vi "Create Execution Unit.vi"(8 "error in":errorcluster, 10 "Item Ref":T2=18446744073709551615 format="%.0x", 11 "Execution Unit Factory Implementation in":refnum<class "Execution Unit Factory.lvclass">) -> (0 "error out":errorcluster, 1 "Asynchronous Execution Units":cluster{"Grouped Execution Units":T1[]}[](array[cluster]) {"Grouped Execution Units"."ReadWrite Channels" format="%.0x"; "Grouped Execution Units"."Outgoing Channels" format="%.0x"; "Grouped Execution Units"."Incoming Channels" format="%.0x"}, 2 "Inline Execution Units":T1[](array[typedef]) {"ReadWrite Channels" format="%.0x"; "Outgoing Channels" format="%.0x"; "Incoming Channels" format="%.0x"}, 3 "Execution Unit Factory Implementation out":refnum<class "Execution Unit Factory.lvclass">)   [LabVIEW 2020, in "Ballard ARINC 429 Engine.lvlib" / "Implementation.lvlib" / "Execution Unit Factory.lvclass"]
uses:
  Execution Unit Factory.lvclass
  <vilib>/NI VeriStand/Custom Device API/Custom Device Item Ref.ctl
  Interfaces/Controls/Execution Unit Information.ctl
  Interfaces/Execution Unit/Execution Unit.lvclass
  Rx Execution Unit/Rx Execution Unit.lvclass
  C:/git/ni/niveristand-ballard-arinc429-custom-device/Source/Custom Device Support/Engine/Interfaces/Execution Unit/Execution Unit.lvclass
  Tx Acyclic Labels Execution Unit/Tx Acyclic Labels Execution Unit.lvclass
  Tx Scheduled Labels Execution Unit/Tx Scheduled Labels Execution Unit.lvclass
  <vilib>/NI VeriStand/Custom Device API/Custom Device API.lvlib
  Interfaces/Interfaces.lvlib
  System Explorer/Implementation/Implementation.lvlib
  Scripting/Ballard/Ballard ARINC 429 Scripting.lvlib
  Custom Device/Custom Device.lvlib
  C:/git/ni/niveristand-ballard-arinc429-custom-device/Source/Custom Device Support/Engine/Implementation/Execution Unit/Execution Unit.lvclass
  C:/git/ni/niveristand-ballard-arinc429-custom-device/Source/Custom Device Support/Engine/Implementation/Rx Execution Unit/Rx Execution Unit.lvclass
  C:/git/ni/niveristand-ballard-arinc429-custom-device/Source/Custom Device Support/Engine/Implementation/Tx Acyclic Labels Execution Unit/Tx Acyclic Labels Execution Unit.lvclass
  C:/git/ni/niveristand-ballard-arinc429-custom-device/Source/Custom Device Support/Engine/Implementation/Tx Scheduled Labels Execution Unit/Tx Scheduled Labels Execution Unit.lvclass
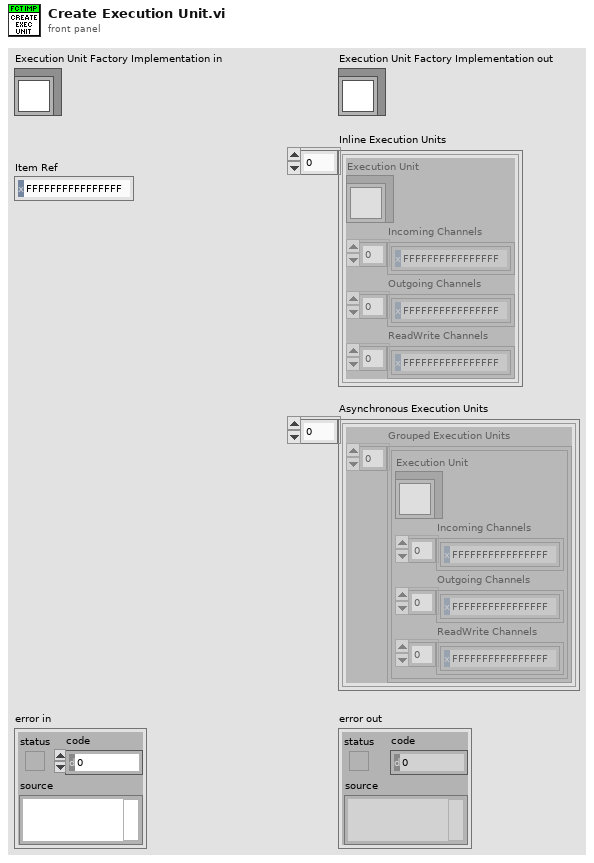
[diagram p1: front panel]
types:
  T1 = typedef "Ballard ARINC 429 Engine.lvlib/Interfaces.lvlib/Execution Unit Information.ctl" = cluster{"Execution Unit":refnum<class "Execution Unit.lvclass">, "Incoming Channels":T2[], "Outgoing Channels":T2[], "ReadWrite Channels":T2[]}
  T2 = typedef "Custom Device API.lvlib/Custom Device Item Ref.ctl" = u64
  T3 = typedef "RT Hardware Channel Settings.ctl" = cluster{"channel #":u16, "channel handle":u64, "labels settings for RT":T4[]}
  T4 = typedef "RT Label Settings.ctl" = cluster{"Name":string, "xmlName":string, "label":T5, "transfer period":u32, "SDI_Enabled":bool, "SDI":u8, "parameter driver data":T6, "transfer type":T9, "has timestamp?":bool, "Label Disable/Trigger Channel Reference":T2, "Message Handle":u64, "Initialized?":bool, "Word Initial Raw Value":u32, "Label Timestamp Channel Data Reference":T10, "disabled":bool}
  T5 = typedef "Label.ctl" = u8
  T6 = typedef "RT Parameters.ctl" = cluster{"parameter definitions":T7[], "Tx parameter refs":T2[]}
  T7 = typedef "Parameter Definition.ctl" = cluster{"start index":i32, "size":i32, "encoding":T8, "signed":bool, "scale multiplier":dbl, "scale offset":dbl}
  T8 = typedef "Encoding and Decoding.lvlib/Encoding.ctl" = enum16{"BNR", "BCD", "Discrete"}
  T9 = typedef "Transfer Type.ctl" = enum16{"Scheduled", "Acyclic", "Block", "Strobe"}
  T10 = typedef "Custom Device API.lvlib/Data Reference.ctl" = i32
  T11 = typedef "Rx Channel Data Offsets.ctl" = cluster{"error counts":u32, "rx execution time":i64}
  T12 = typedef "Custom Device API.lvlib/Custom Device Item Info.ctl" = cluster{"Name":string, "Is Channel":bool, "GUID":string, "Is Waveform":bool}
  T13 = cluster{"transfer type":T9, "Name":string, "hardware channel data":T3[], "Outgoing Channels":T2[], "ReadWrite Channels":T2[]}[]
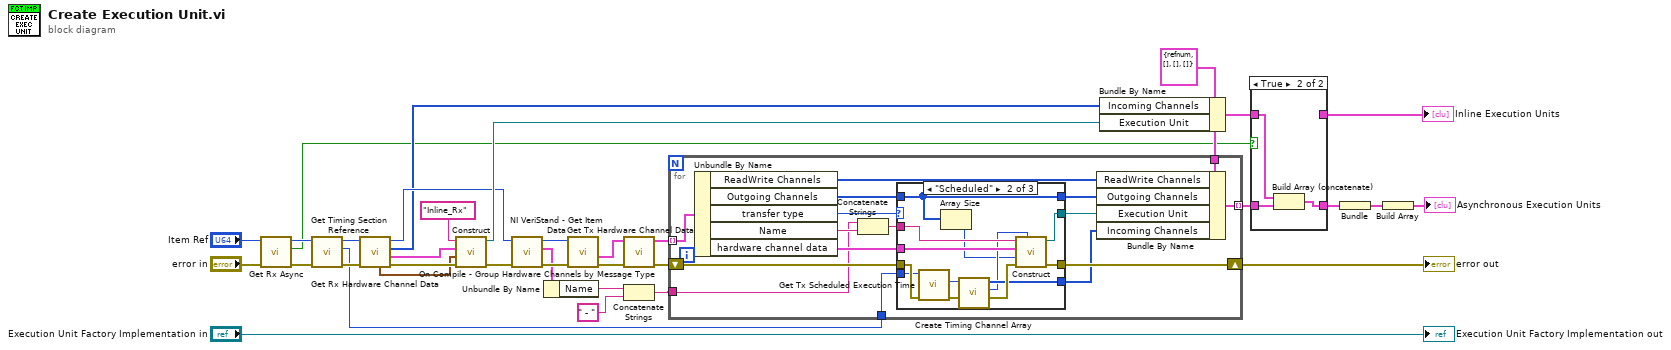
[diagram p0: block diagram]
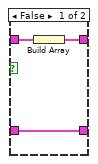
[diagram p2: hidden frame]
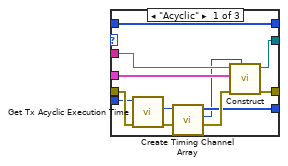
[diagram p3: hidden frame]
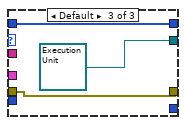
[diagram p4: hidden frame]
diagram:
  w23 = T1 {"Execution Unit"=refnum, "Incoming Channels"=[], "Outgoing Channels"=[], "ReadWrite Channels"=[]} ("Execution Unit Information")
  n1 = call "Get Rx Async.vi"("error in"="error in", "Ballard ARINC 429 custom device in"="Item Ref") -> ("error out"=w7:errorcluster, "rx async?"=w5:bool, "Ballard ARINC 429 custom device out"=w8:T2)  [unwired: 7 in]
  n2 = call "Get Timing Section Reference.vi"("error in"=w7, "Ballard ARINC 429 ref"=w8) -> ("error out"=w12:errorcluster, "timing section ref"=w9:T2, "Ballard ARINC 429 ref out"=w11:T2)  [unwired: 6 in, 1 out]
  n3 = call "Get Rx Hardware Channel Data.vi"("error in"=w12, "custom device ref in"=w11) -> ("error out"=w28:errorcluster, "Rx hardware channel data"=w29:T3[], "incoming channels"=w14:T2[], "custom device ref out"=w21:T2, "channel data offsets"=w13:T11)  [unwired: 5 in]
  n4 = call "Construct.vi"("error in"=w28, "channel data offsets"=w13, "RT hardware channels"=w29, "ID"="Inline_Rx") -> ("error out"=w22:errorcluster, "Ballard ARINC-429 Rx Execution Unit"=w27:refnum<class "Rx Execution Unit.lvclass">)  [unwired: 6 in]
  n5 = call <vilib>:"NI VeriStand - Get Item Data.vi"("error in (no error)"=w22, "Item Ref in"=w21) -> ("error out"=w19:errorcluster, "Item Info"=w18:T12, "Item Ref out"=w20:T2)  [unwired: 6 in, 1 out]
  n6 = Unbundle By Name(w18) -> ("Name"=w17:string)
  n7 = call "Get Tx Hardware Channel Data.vi"("error in"=w19, "custom device ref in"=w20) -> ("error out"=w31:errorcluster, "Tx hardware channel data"=w30:T3[])  [unwired: 6 in, 2 out]
  n8 = call "On Compile - Group Hardware Channels by Message Type.vi"("error in"=w31, "hardware channel data"=w30) -> ("error out"=w26:errorcluster, "hardware channel data by transfer type"=w24:T13)  [unwired: 8 in]
  n9 = Concatenate Strings(w17, " - " ("string")) -> (w15:string)
  n10 = for {
    shift-right: [w50] -> w25
    shift-left: w26 -> [w51]
    tunnel: w24 -> [w49] mode=indexing
    tunnel: w23 -> [w47]
    tunnel: [w45] -> w2 mode=indexing
    tunnel: w15 -> [w41]
    tunnel: w9 -> [w39]
    n11 = Unbundle By Name(w49) -> ("ReadWrite Channels"=w44:T2[], "Outgoing Channels"=w37:T2[], "transfer type"=w46:T9, "Name"=w42:string, "hardware channel data"=w43:T3[])
    n12 = Concatenate Strings(w41, w42) -> (w40:string)
    n13 = case shown="\"Scheduled\"" w46 {
      tunnel: w43 -> [w62 w74 _]
      tunnel: [w61 w73 refnum<class "Execution Unit.lvclass"> refnum ("Execution Unit")] -> w48
      tunnel: w51 -> [w58 w70 w76]
      tunnel: [w60 w72 w76] -> w50
      tunnel: w40 -> [w59 w71 _]
      tunnel: w39 -> [w57 w69 _]
      tunnel: [w54 w66 _] -> w38
      tunnel: w37 -> [w52 w64 w75]
      tunnel: [w52 w64 w75] -> w36
      frame "Acyclic" {
        n14 = call "Get Tx Acyclic Execution Time.vi"("error in"=w58, "timing section in"=w57) -> ("error out"=w56:errorcluster, "tx acyclic execution time ref"=w55:T2)  [unwired: 7 in, 1 out]
        n15 = call "Create Timing Channel Array.vi"("timing channel ref"=w55) -> ("channel offset"=w53:i64, "timing channel ref array"=w54:T2[])  [unwired: 9 in]
        n16 = call "Construct.vi"("timing channel offset"=w53, "error in"=w56, "RT hardware channels"=w62, "ID"=w59) -> ("error out"=w60:errorcluster, "Ballard ARINC-429 Tx Acyclic execution unit out"=w61:refnum<class "Tx Acyclic Labels Execution Unit.lvclass">)  [unwired: 6 in]
      }
      frame "Scheduled" {
        n17 = call "Get Tx Scheduled Execution Time.vi"("error in"=w70, "timing section in"=w69) -> ("error out"=w68:errorcluster, "tx scheduled execution time ref"=w67:T2)  [unwired: 7 in, 1 out]
        n18 = Array Size(array=w64) -> (size(s)=w63:i32)
        n19 = call "Create Timing Channel Array.vi"("timing channel ref"=w67) -> ("channel offset"=w65:i64, "timing channel ref array"=w66:T2[])  [unwired: 9 in]
        n20 = call "Construct.vi"("timing channel offset"=w65, "error in"=w68, "outgoing channel count"=w63, "RT hardware channels"=w74, "ID"=w71) -> ("error out"=w72:errorcluster, "Ballard ARINC-429 Tx Execution Unit out"=w73:refnum<class "Tx Scheduled Labels Execution Unit.lvclass">)  [unwired: 5 in]
      }
      frame Default {
      }
    }
    n21 = Bundle By Name(cluster=w47, "ReadWrite Channels"=w44, "Outgoing Channels"=w36, "Execution Unit"=w48, "Incoming Channels"=w38) -> (w45:T1)
  }
  "error out" <- w25
  n22 = Bundle By Name(cluster=w23, "Incoming Channels"=w14, "Execution Unit"=w27) -> (w34:T1)
  n23 = case shown="True" w5 {
    tunnel: w34 -> [w80 w82]
    tunnel: [w79 _] -> w33
    tunnel: w2 -> [w78 w83]
    tunnel: [w78 w81] -> w1
    frame False {
      n24 = Build Array(w80) -> (w79:T1[])
    }
    frame True {
      n25 = Build Array (concatenate)(w82, w83) -> (w81:T1[])
    }
  }
  "Inline Execution Units" <- w33
  n26 = Bundle(w1) -> (w4:cluster{T1[]})  [unwired: 1 in]
  n27 = Build Array(w4) -> (→"Asynchronous Execution Units":cluster{T1[]}[])
  "Execution Unit Factory Implementation out" <- "Execution Unit Factory Implementation in"
